vi "Actor Core.vi"(8 "error in":errorcluster, 11 "Configuration Window in":refnum<class "Configuration Window.lvclass">) -> (0 "error out":errorcluster, 3 "Actor out":refnum<class "Actor.lvclass">)   [LabVIEW 2018, in "Configuration Window.lvlib" / "Configuration Window.lvclass"]
doc: "The user interface for this panel.\n\n----\nPlease see the following web address for additional documentation and tutorial information:\nhttp://www.mooregoodideas.com/mgi-panel-manager/\n\nAuthor: Derek Trepanier\n\nCopyright (c) 2018, Moore Good Ideas, Inc.\n\nAll rights reserved.\n\nRedistribution and use in source and binary forms, with or without modification, are permitted provided that the following conditions are met:\n\n * Redistributions of source code must retain the above copyright notice, this list of conditions and the following disclaimer.\n * Redistributions in binary form must reproduce the above copyright notice, this list of conditions and the following disclaimer in the documentation and/or other materials provided with the distribution.\n * Neither the name of Moore Good Ideas, Inc. nor the names of its contributors may be used to endorse or promote products derived from this software without specific prior written permission.\n\nTHIS SOFTWARE IS PROVIDED BY THE COPYRIGHT HOLDERS AND CONTRIBUTORS \"AS IS\" AND ANY EXPRESS OR IMPLIED WARRANTIES, INCLUDING, BUT NOT LIMITED TO, THE IMPLIED WARRANTIES OF MERCHANTABILITY AND FITNESS FOR A PARTICULAR PURPOSE ARE DISCLAIMED. IN NO EVENT SHALL THE COPYRIGHT OWNER OR CONTRIBUTORS BE LIABLE FOR ANY DIRECT, INDIRECT, INCIDENTAL, SPECIAL, EXEMPLARY, OR CONSEQUENTIAL DAMAGES (INCLUDING, BUT NOT LIMITED TO, PROCUREMENT OF SUBSTITUTE GOODS OR SERVICES; LOSS OF USE, DATA, OR PROFITS; OR BUSINESS INTERRUPTION) HOWEVER CAUSED AND ON ANY THEORY OF LIABILITY, WHETHER IN CONTRACT, STRICT LIABILITY, OR TORT (INCLUDING NEGLIGENCE OR OTHERWISE) ARISING IN ANY WAY OUT OF THE USE OF THIS SOFTWARE, EVEN IF ADVISED OF THE POSSIBILITY OF SUCH DAMAGE."
uses:
  Configuration Window.lvclass
  C:/Program Files (x86)/National Instruments/LabVIEW 2018/vi.lib/MGI/Panel Manager/Panel Actor/Panel Actor/Panel Actor.lvclass
  <vilib>/ActorFramework/Actor/Actor.lvclass
  Configuration Window.lvclass/Configuration Window.ctl
  Framework/Framework/Framework.lvclass
  <vilib>/MGI/Panel Manager/Panel Actor/Panel Actor/Panel Actor.lvclass
panel:
  in  "Cancel":bool
  in  "Save":bool
  in  "Tab Control":enum32{"Main", "Image"}(tab)
  in  "Language":u16(ring)
  in  "_res_pngs Folder Path":path
  in  "_res_data Folder Path":path
  in  "Reset to Steam Path":bool
  out "c Name":string="<c> Point:"
  out "o Name":string="<o> Point:"
  out "i Name":string="<i> Box:"
  out "b Name":string="<b> Box:"
  out "w Name":string="<w> Point:"
  out "bp Name":string="<bp> Point:"
  in  "c Size":i32 caption="Size"
  in  "c Enable":bool caption="Enable"
  in  "c Color":u32(colorbox) caption="Color"
  in  "o Size":i32 caption="Size"
  in  "o Enable":bool caption="Enable"
  in  "o Color":u32(colorbox) caption="Color"
  in  "i Fill Color":u32(colorbox) caption="Fill Color"
  in  "i Enable":bool caption="Enable"
  in  "i Border Color":u32(colorbox) caption="Border Color"
  in  "b Fill Color":u32(colorbox) caption="Fill Color"
  in  "b Enable":bool caption="Enable"
  in  "b Border Color":u32(colorbox) caption="Border Color"
  in  "w Enable":bool caption="Enable"
  in  "w Color":u32(colorbox) caption="Color"
  in  "w Size":i32 caption="Size"
  in  "bp Enable":bool caption="Enable"
  in  "bp Color":u32(colorbox) caption="Color"
  in  "bp Size":i32 caption="Size"
  in  "CP Enable":bool caption="Enable"
  in  "CP Color":u32(colorbox) caption="Color"
  in  "CP Size":i32 caption="Size"
  out "CP Name":string="Center Point:"
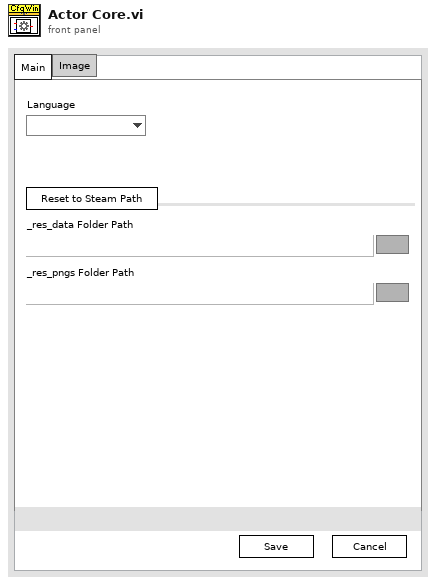
[diagram p1: front panel]
types:
  T1 = cluster{"Reset to Steam Path":refnum<vi>, "_res_data Folder Path":refnum<vi>, "_res_pngs Folder Path":refnum<vi>}
  T2 = cluster{"CP Name":refnum<vi>, "CP Size":refnum<vi>, "CP Color":refnum<vi>, "CP Enable":refnum<vi>}
  T3 = cluster{"bp Name":refnum<vi>, "bp Size":refnum<vi>, "bp Color":refnum<vi>, "bp Enable":refnum<vi>}
  T4 = cluster{"w Name":refnum<vi>, "w Size":refnum<vi>, "w Color":refnum<vi>, "w Enable":refnum<vi>}
  T5 = cluster{"b Name":refnum<vi>, "b Fill Color":refnum<vi>, "b Border Color":refnum<vi>, "b Enable":refnum<vi>}
  T6 = cluster{"i Name":refnum<vi>, "i Fill Color":refnum<vi>, "i Border Color":refnum<vi>, "i Enable":refnum<vi>}
  T7 = cluster{"o Name":refnum<vi>, "o Size":refnum<vi>, "o Color":refnum<vi>, "o Enable":refnum<vi>}
  T8 = cluster{"c Name":refnum<vi>, "c Size":refnum<vi>, "c Color":refnum<vi>, "c Enable":refnum<vi>}
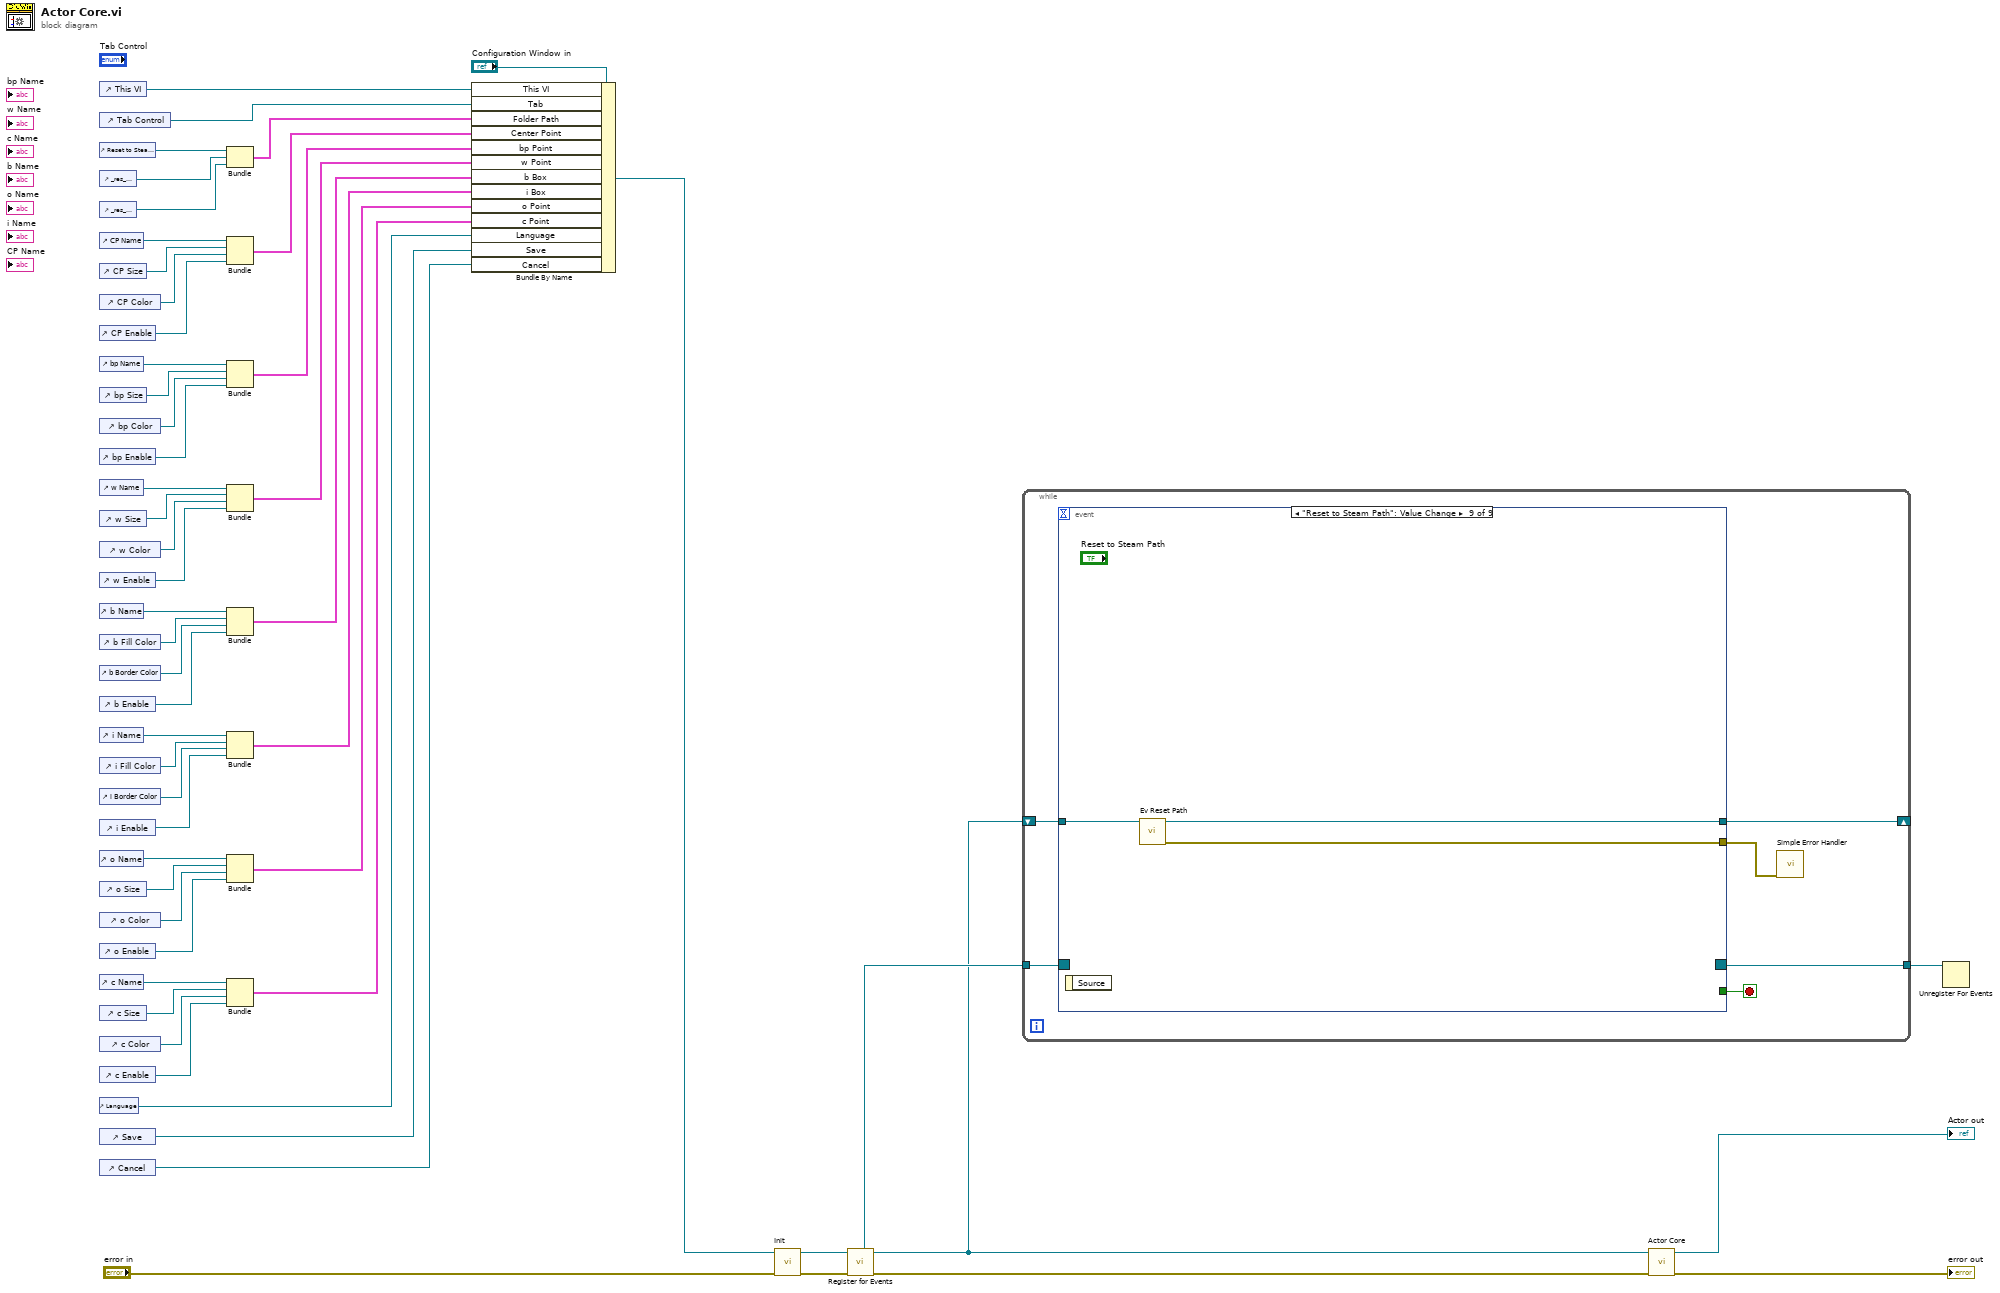
[diagram p0: block diagram]
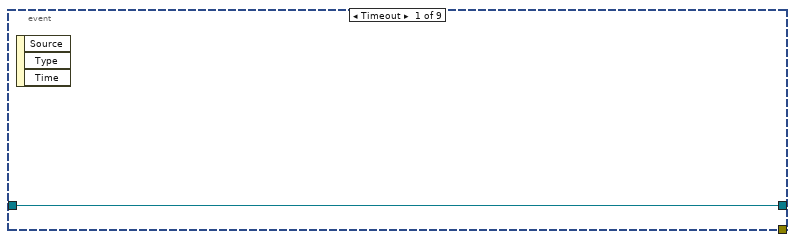
[diagram p2: hidden frame]
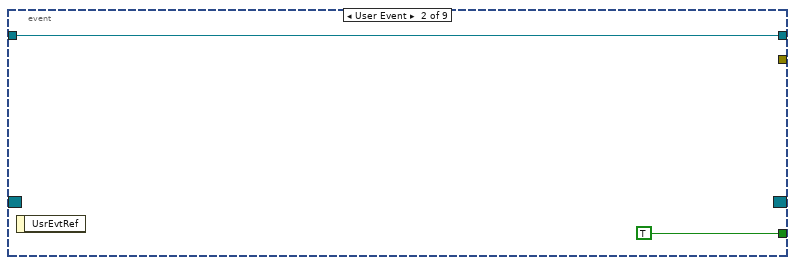
[diagram p3: hidden frame]
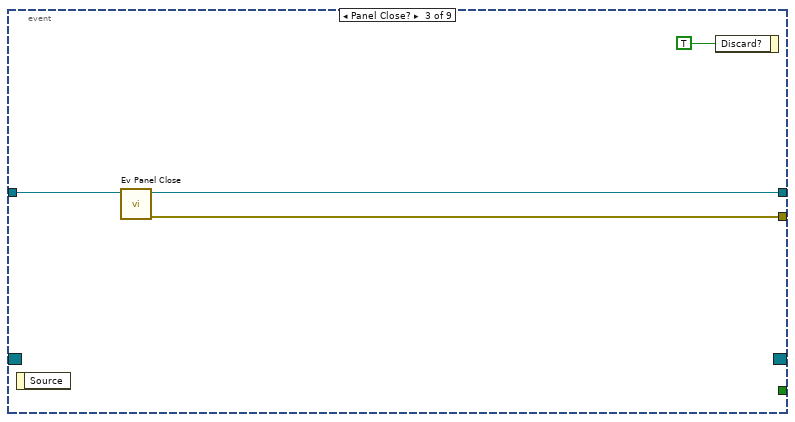
[diagram p4: hidden frame]
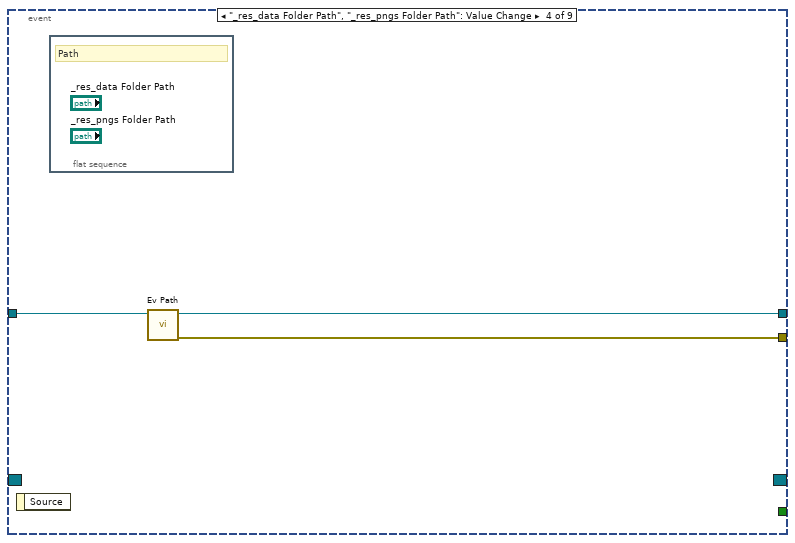
[diagram p5: hidden frame]
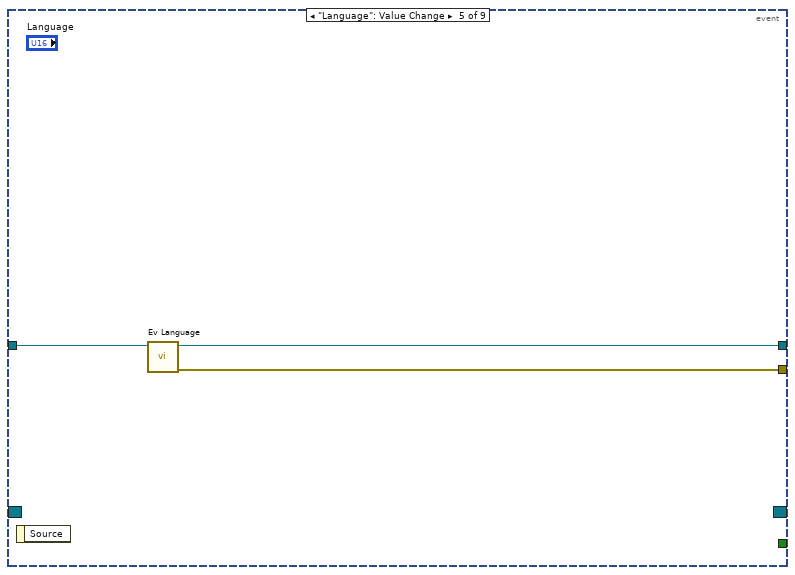
[diagram p6: hidden frame]
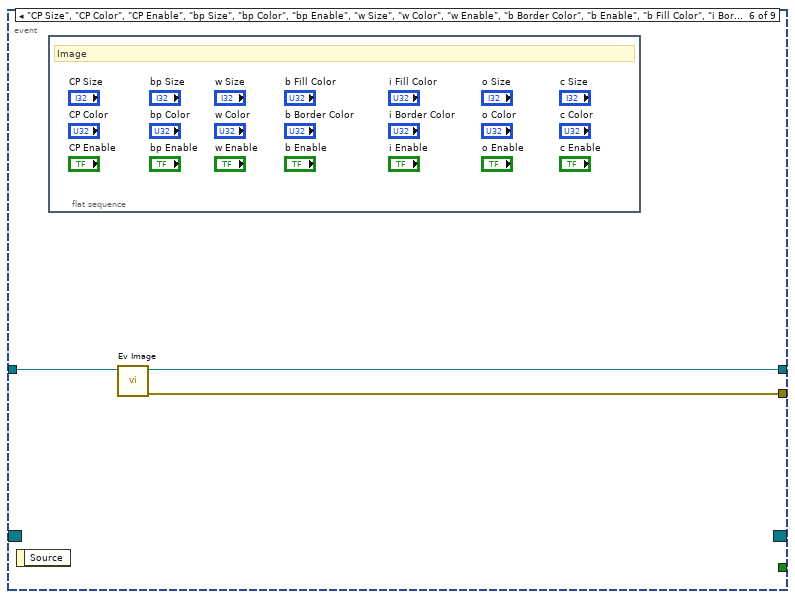
[diagram p7: hidden frame]
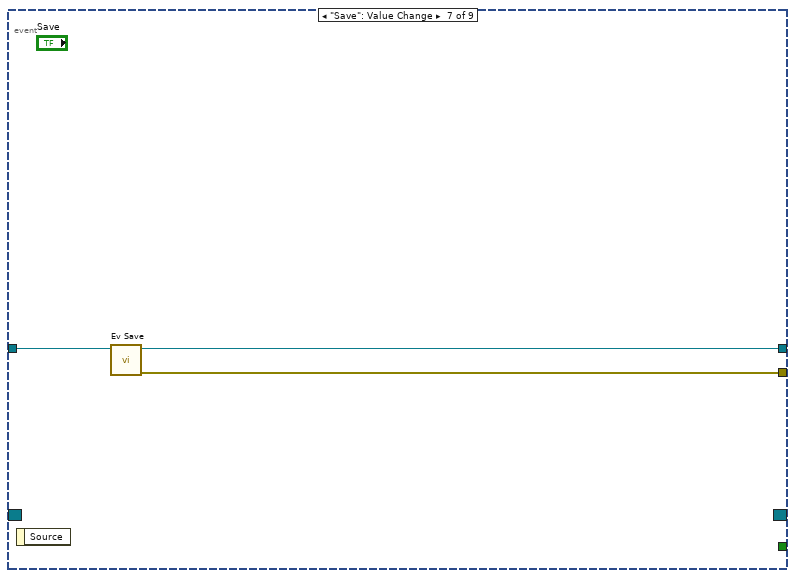
[diagram p8: hidden frame]
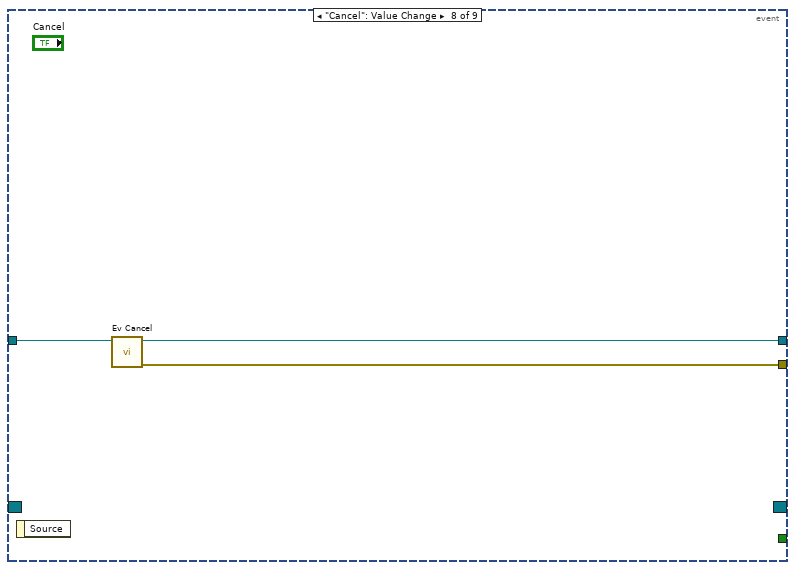
[diagram p9: hidden frame]
diagram:
  n1 = control-ref of="This VI"() -> (w48:refnum<vi>)
  n2 = control-ref of="Tab Control"() -> (w4:refnum<vi>)
  n3 = control-ref of="Reset to Steam Path"() -> (w1:refnum<vi>)
  n4 = control-ref of="_res_data Folder Path"() -> (w47:refnum<vi>)
  n5 = control-ref of="_res_pngs Folder Path"() -> (w46:refnum<vi>)
  n6 = control-ref of="CP Name"() -> (w5:refnum<vi>)
  n7 = control-ref of="CP Size"() -> (w44:refnum<vi>)
  n8 = control-ref of="CP Color"() -> (w43:refnum<vi>)
  n9 = control-ref of="CP Enable"() -> (w42:refnum<vi>)
  n10 = control-ref of="bp Name"() -> (w6:refnum<vi>)
  n11 = control-ref of="bp Size"() -> (w40:refnum<vi>)
  n12 = control-ref of="bp Color"() -> (w39:refnum<vi>)
  n13 = control-ref of="bp Enable"() -> (w38:refnum<vi>)
  n14 = control-ref of="w Name"() -> (w7:refnum<vi>)
  n15 = control-ref of="w Size"() -> (w36:refnum<vi>)
  n16 = control-ref of="w Color"() -> (w35:refnum<vi>)
  n17 = control-ref of="w Enable"() -> (w34:refnum<vi>)
  n18 = control-ref of="b Name"() -> (w8:refnum<vi>)
  n19 = control-ref of="b Fill Color"() -> (w32:refnum<vi>)
  n20 = control-ref of="b Border Color"() -> (w31:refnum<vi>)
  n21 = control-ref of="b Enable"() -> (w30:refnum<vi>)
  n22 = control-ref of="i Name"() -> (w9:refnum<vi>)
  n23 = control-ref of="i Fill Color"() -> (w28:refnum<vi>)
  n24 = control-ref of="i Border Color"() -> (w27:refnum<vi>)
  n25 = control-ref of="i Enable"() -> (w26:refnum<vi>)
  n26 = control-ref of="o Name"() -> (w10:refnum<vi>)
  n27 = control-ref of="o Size"() -> (w24:refnum<vi>)
  n28 = control-ref of="o Color"() -> (w23:refnum<vi>)
  n29 = control-ref of="o Enable"() -> (w22:refnum<vi>)
  n30 = control-ref of="c Name"() -> (w11:refnum<vi>)
  n31 = control-ref of="c Size"() -> (w20:refnum<vi>)
  n32 = control-ref of="c Color"() -> (w19:refnum<vi>)
  n33 = control-ref of="c Enable"() -> (w18:refnum<vi>)
  n34 = control-ref of="Language"() -> (w12:refnum<vi>)
  n35 = control-ref of="Save"() -> (w3:refnum<vi>)
  n36 = control-ref of="Cancel"() -> (w2:refnum<vi>)
  n37 = Bundle("Reset to Steam Path"=w1, "_res_data Folder Path"=w47, "_res_pngs Folder Path"=w46) -> (w45:T1)  [unwired: 1 in]
  n38 = Bundle("CP Name"=w5, "CP Size"=w44, "CP Color"=w43, "CP Enable"=w42) -> (w41:T2)  [unwired: 1 in]
  n39 = Bundle("bp Name"=w6, "bp Size"=w40, "bp Color"=w39, "bp Enable"=w38) -> (w37:T3)  [unwired: 1 in]
  n40 = Bundle("w Name"=w7, "w Size"=w36, "w Color"=w35, "w Enable"=w34) -> (w33:T4)  [unwired: 1 in]
  n41 = Bundle("b Name"=w8, "b Fill Color"=w32, "b Border Color"=w31, "b Enable"=w30) -> (w29:T5)  [unwired: 1 in]
  n42 = Bundle("i Name"=w9, "i Fill Color"=w28, "i Border Color"=w27, "i Enable"=w26) -> (w25:T6)  [unwired: 1 in]
  n43 = Bundle("o Name"=w10, "o Size"=w24, "o Color"=w23, "o Enable"=w22) -> (w21:T7)  [unwired: 1 in]
  n44 = Bundle("c Name"=w11, "c Size"=w20, "c Color"=w19, "c Enable"=w18) -> (w17:T8)  [unwired: 1 in]
  n45 = Bundle By Name(cluster="Configuration Window in", "This VI"=w48, "Tab"=w4, "Folder Path"=w45, "Center Point"=w41, "bp Point"=w37, "w Point"=w33, "b Box"=w29, "i Box"=w25, "o Point"=w21, "c Point"=w17, "Language"=w12, "Save"=w3, "Cancel"=w2) -> (w16:refnum<class "Configuration Window.lvclass">)
  n46 = call "Init.vi"("error in (no error)"="error in", "Configuration Window in"=w16) -> ("error out"=w14:errorcluster, "Configuration Window out"=w15:refnum<class "Configuration Window.lvclass">)  [unwired: 8 in]
  n47 = call <vilib>:"Register for Events.vi"("Error In"=w14, "Panel Actor in"=w15) -> ("Error Out"=w52:errorcluster, "Panel Actor out"=w50:refnum<class "Configuration Window.lvclass">, "Pnl Actor"=w51:refnum<event-registration>)  [unwired: 6 in, 1 out]
  n48 = while {
    tunnel: [w60] -> w53
    tunnel: w51 -> [w59]
    shift-right: [w57] -> _
    shift-left: w50 -> [w58]
    stop <- w61 stop-if-true
    n49 = event shown="[8] \"Reset to Steam Path\": Value Change" {
      selector: w59 -> [_ _ _ _ _ _ _ _ _]
      dyn-events: [_ _ _ _ _ _ _ _ _] -> w60
      timeout: _ -> [_ _ _ _ _ _ _ _ _]
      tunnel: [_ TRUE _ _ _ _ _ _ _] -> w61
      tunnel: w58 -> [w62 w63 w67 w71 w74 w77 w80 w83 w86]
      tunnel: [w62 w63 w65 w69 w72 w76 w78 w81 w84] -> w57
      tunnel: [_ _ w66 w70 w73 w75 w79 w82 w85] -> w56
      event Timeout {
        n50 = event-data() -> ()  [unwired: 1 in, 3 out]
      }
      event User Event {
        n51 = event-data() -> ()  [unwired: 1 in, 1 out]
      }
      event Panel Close? {
        n52 = event-data() -> ()  [unwired: 1 in, 1 out]
        n53 = call "Ev Panel Close.vi"("Configuration Window in"=w67) -> ("error out"=w66:errorcluster, "Configuration Window out"=w65:refnum<class "Configuration Window.lvclass">)  [unwired: 9 in]
        n54 = event-data("Discard?"=TRUE) -> ()  [unwired: 1 in, 1 out]
      }
      event "_res_data Folder Path", "_res_pngs Folder Path": Value Change {
        n55 = event-data() -> ()  [unwired: 1 in, 1 out]
        n56 = flat-sequence {
          frame #0 {
            # "Path"
          }
        }
        n57 = call "Ev Path.vi"("Configuration Window in"=w71) -> ("error out"=w70:errorcluster, "Configuration Window out"=w69:refnum<class "Configuration Window.lvclass">)  [unwired: 9 in]
      }
      event "Language": Value Change {
        n58 = event-data() -> ()  [unwired: 1 in, 1 out]
        n59 = call "Ev Language.vi"("Configuration Window in"=w74) -> ("error out"=w73:errorcluster, "Configuration Window out"=w72:refnum<class "Configuration Window.lvclass">)  [unwired: 9 in]
      }
      event "CP Size", "CP Color", "CP Enable", "bp Size", "bp Color", "bp Enable", "w Size", "w Color", "w Enable", "b Border Color", "b Enable", "b Fill Color", "i Border Color", "i Enable", "i Fill Color", "o Color", "o Enable", "o Size", "c Color", "c Enable", "c Size": Value Change {
        n60 = event-data() -> ()  [unwired: 1 in, 1 out]
        n61 = flat-sequence {
          frame #0 {
            # "Image"
          }
        }
        n62 = call "Ev Image.vi"("Configuration Window in"=w77) -> ("error out"=w75:errorcluster, "Configuration Window out"=w76:refnum<class "Configuration Window.lvclass">)  [unwired: 9 in]
      }
      event "Save": Value Change {
        n63 = event-data() -> ()  [unwired: 1 in, 1 out]
        n64 = call "Ev Save.vi"("Configuration Window in"=w80) -> ("error out"=w79:errorcluster, "Configuration Window out"=w78:refnum<class "Configuration Window.lvclass">)  [unwired: 9 in]
      }
      event "Cancel": Value Change {
        n65 = event-data() -> ()  [unwired: 1 in, 1 out]
        n66 = call "Ev Cancel.vi"("Configuration Window in"=w83) -> ("error out"=w82:errorcluster, "Configuration Window out"=w81:refnum<class "Configuration Window.lvclass">)  [unwired: 9 in]
      }
      event "Reset to Steam Path": Value Change {
        n67 = event-data() -> ()  [unwired: 1 in, 1 out]
        n68 = call "Ev Reset Path.vi"("Configuration Window in"=w86) -> ("error out"=w85:errorcluster, "Configuration Window out"=w84:refnum<class "Configuration Window.lvclass">)  [unwired: 9 in]
      }
    }
    n69 = call <vilib>:"Simple Error Handler.vi"("error in (no error)"=w56) -> ()  [unwired: 4 in, 5 out]
  }
  n70 = call-parent "Actor Core.vi"("error in"=w52, "Panel Actor in"=w50) -> ("error out"=→"error out":errorcluster, "Actor out"=→"Actor out":refnum<class "Actor.lvclass">)  [unwired: 8 in]
  n71 = Unregister For Events(event registration refnum=w53) -> ()  [unwired: 1 in, 1 out]
